vi "initAppLayerCmdFile.vi"   [LabVIEW 2010]
uses:
  <vilib>/xml/Load XML File.vi
  AmmeterGlobalCostants.vi
  <vilib>/xml/NI_XML.lvlib
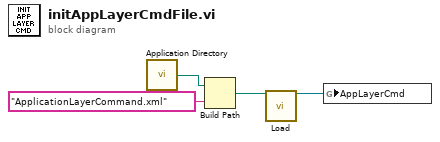
[diagram p0: block diagram]
diagram:
  n1 = call <vilib>:"Application Directory.vi"() -> ("Application Directory"=w4:path)
  n2 = Build Path(base path=w4, name or relative path="ApplicationLayerCommand.xml") -> (appended path=w2:path)
  n3 = call-poly <vilib>:"Load.vi"("path to XML document"=w2) -> ("DOM document out"=w1:refnum<k20>)  [unwired: 12 in, 2 out]
  n4 = global write "AmmeterGlobalCostants.vi" "AppLayerCmd"(w1) -> ()
